vi "AI@SegmentEditor__Parameter.vi"(1 "ParamterIn":string) -> (0 "ParamterOut":string)   [LabVIEW 2020]
uses:
  MainFrame/Global.vi
  <vilib>/vision/NI_Vision_Development_Module.lvlib
panel:
  out "Image":T1(plugin-control)
  in  "Preview":bool
  in  "SubDir":string(combo)
  in  "Capture":string(combo)
  in  "Confirm":bool
  # "AI@SegmentEditor $Capture(\\$Directory)"
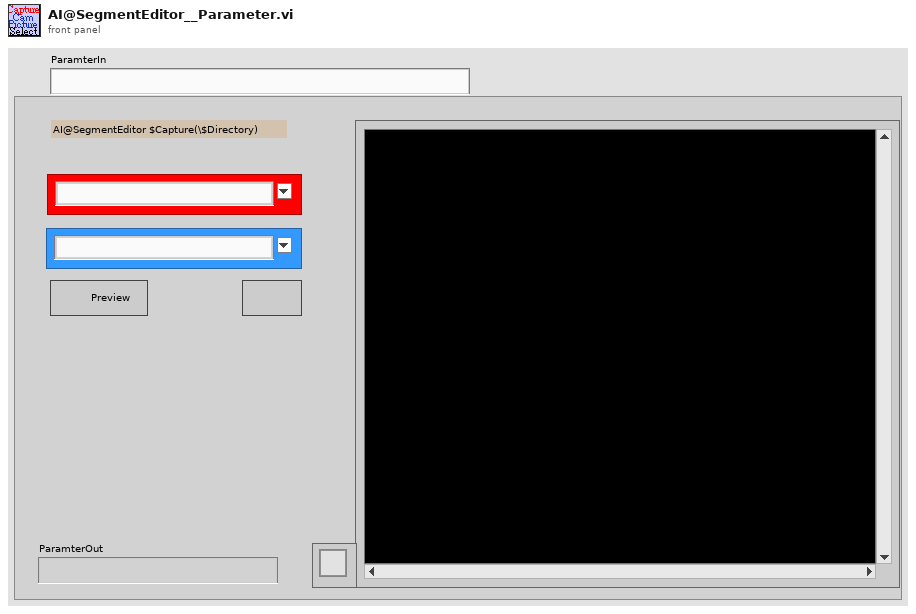
[diagram p1: front panel]
types:
  T1 = typedef "IMAQ Image.ctl" = refnum<image>
  T2 = cluster{"Browser Size":cluster{"X":i32, "Y":i32}, "Images per Line":i32, "Background Color":u32, "Frame Size":i32, "Frame Style":u16}
  T3 = typedef "Image Type" = u32
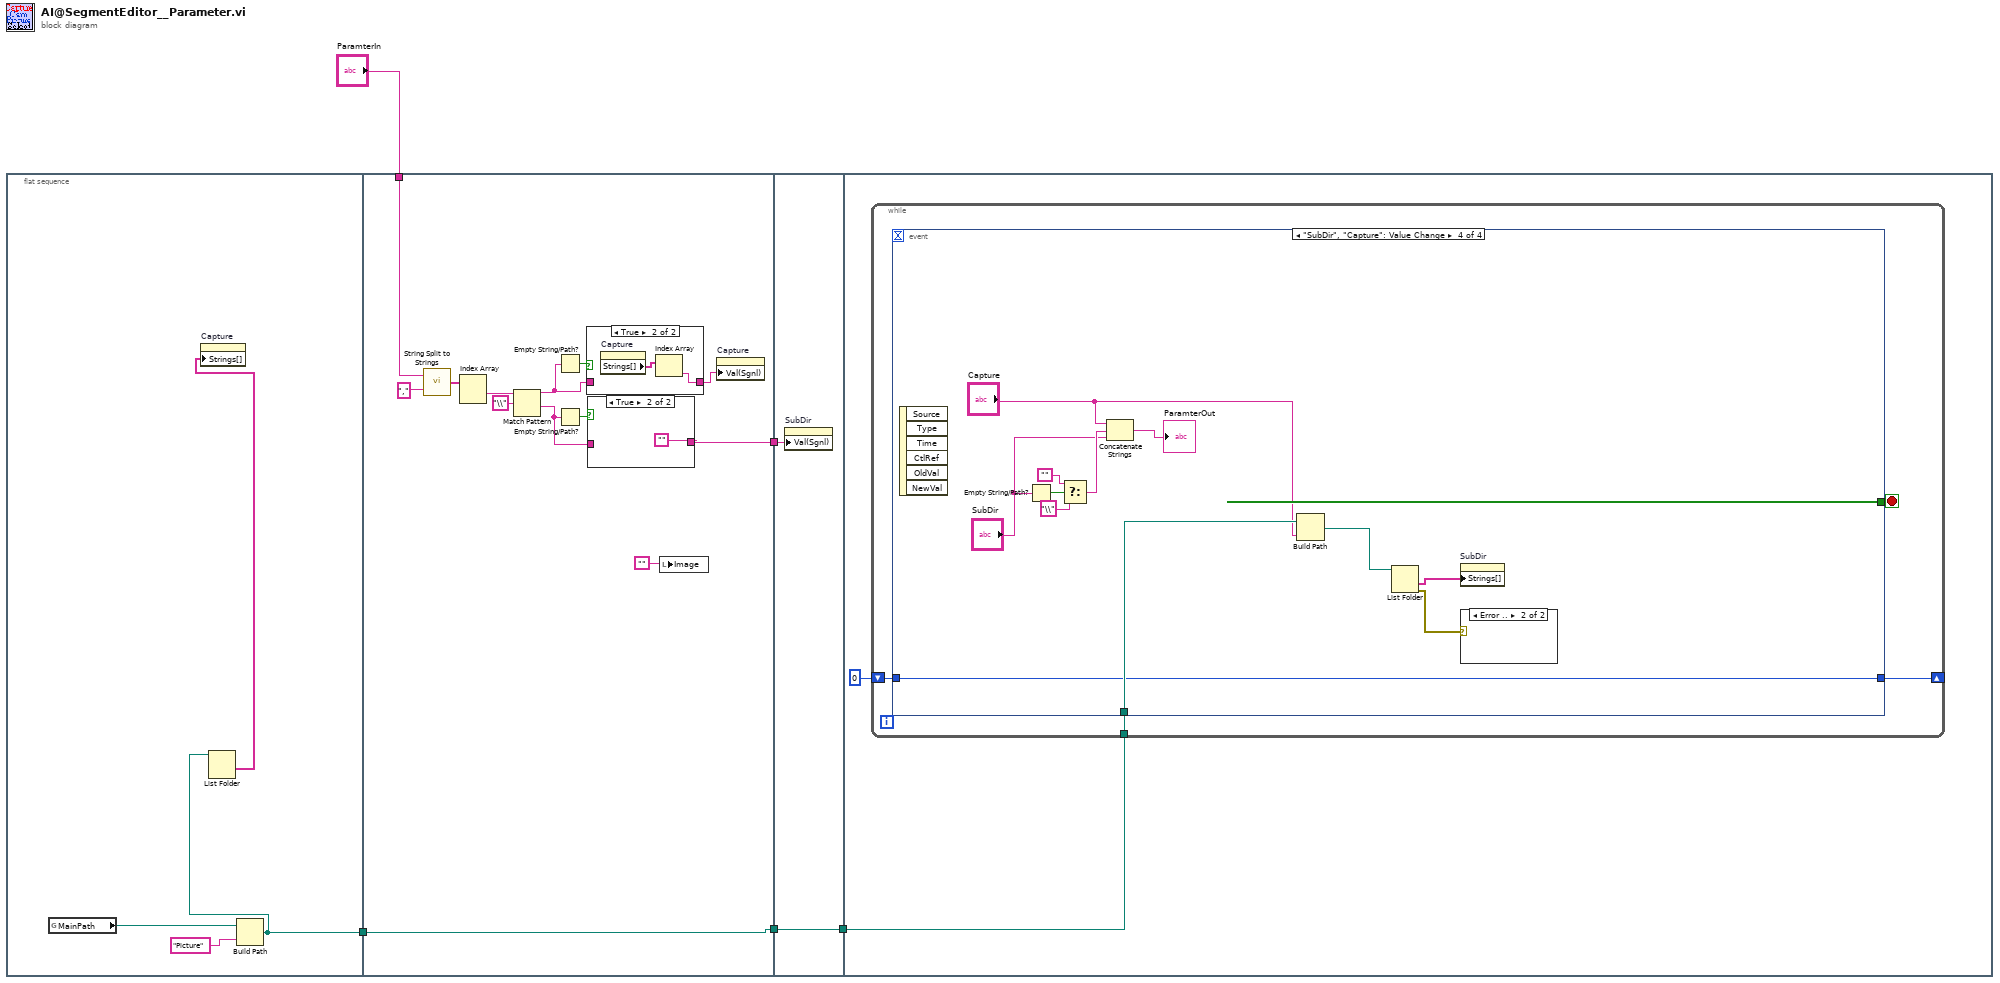
[diagram p0: block diagram]
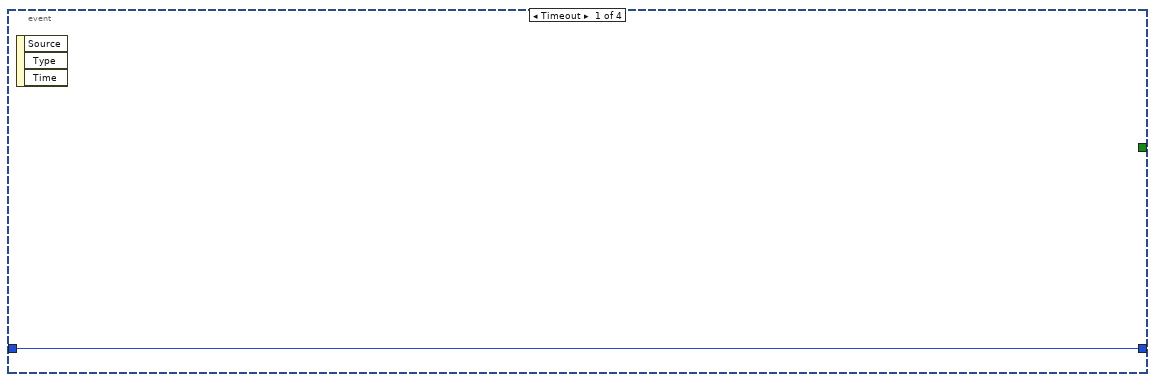
[diagram p4: hidden frame]
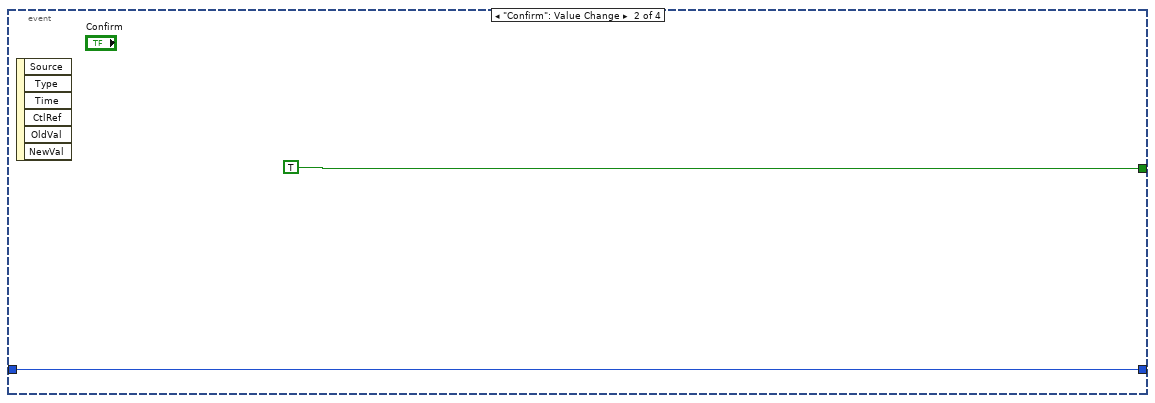
[diagram p5: hidden frame]
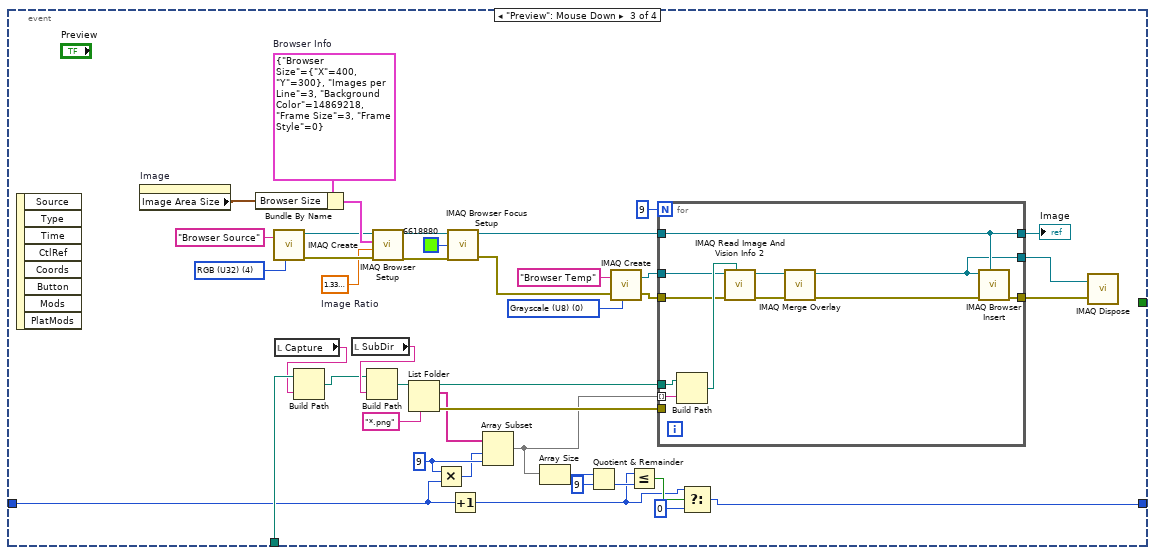
[diagram p6: hidden frame]
diagram:
  n1 = flat-sequence {
    tunnel: [w7] -> w2
    tunnel: "ParamterIn" -> [w20]
    tunnel: [w18] -> w3
    tunnel: w2 -> [w18]
    tunnel: [w17] -> w1
    tunnel: [w29] -> w4
    tunnel: w3 -> [w29]
    tunnel: w1 -> [w28]
    tunnel: w4 -> [w31]
    frame #0 {
      n2 = global read "Global.vi" "MainPath"() -> (w8:path)
      n3 = Build Path(base path=w8, name or relative path="Picture") -> (appended path=w7:path)
      n4 = List Folder(path=w7) -> (folder names=w6:string[])  [unwired: 3 in, 3 out]
      n5 = property on="Capture" class="CmbBox"("Strings[]"=w6) -> ()  [unwired: 2 in, 2 out]
    }
    frame #1 {
      n6 = call "String Split to Strings.vi"("search string/char (-)"=",", "String"=w20) -> ("Array"=w22:string[])
      n7 = Index Array(array=w22) -> (element #1=w14:string)  [unwired: 2 in, 1 out]
      n8 = Match Pattern(string=w14, regular expression="\\") -> (before substring=w12:string, after substring=w11:string)  [unwired: 1 in, 2 out]
      n9 = Empty String/Path?(string/path=w12) -> (empty?=w19:bool)
      n10 = Empty String/Path?(string/path=w11) -> (empty?=w15:bool)
      n11 = case shown="True" w19 {
        tunnel: w12 -> [w25 _]
        tunnel: [w25 w26] -> w16
        frame False {
        }
        frame True {
          n12 = property on="Capture" class="CmbBox"() -> ("Strings[]"=w27:string[])  [unwired: 2 in, 2 out]
          n13 = Index Array(array=w27) -> (element=w26:string)  [unwired: 1 in]
        }
      }
      n14 = case shown="True" w15 {
        tunnel: [w23 ""] -> w17
        tunnel: w11 -> [w23 _]
        frame False {
        }
        frame True {
        }
      }
      n15 = local write "Image"("") -> ()
      n16 = property on="Capture" class="CmbBox"("Val(Sgnl)"=w16) -> ()  [unwired: 2 in, 2 out]
    }
    frame #2 {
      n17 = property on="SubDir" class="CmbBox"("Val(Sgnl)"=w28) -> ()  [unwired: 2 in, 2 out]
    }
    frame #3 {
      n18 = while {
        tunnel: w31 -> [w34]
        shift-right: [w32] -> _
        shift-left: 0 -> [w33]
        stop <- w35 stop-if-true
        n19 = event shown="[3] \"SubDir\", \"Capture\": Value Change" {
          selector: _ -> [_ _ _ _]
          dyn-events: _ -> [_ _ _ _]
          timeout: _ -> [_ _ _ _]
          tunnel: [_ TRUE _ _] -> w35
          tunnel: w34 -> [_ _ w54 w100]
          tunnel: w33 -> [w36 w37 w48 w91]
          tunnel: [w36 w37 w40 w91] -> w32
          event Timeout {
            n20 = event-data() -> ()  [unwired: 1 in, 3 out]
          }
          event "Confirm": Value Change {
            n21 = event-data() -> ()  [unwired: 1 in, 6 out]
          }
          event "Preview": Mouse Down {
            w50 = 9 ("length")
            w58 = sgl 1.33  # Image Ratio
            w75 = T2 {"Browser Size"={"X"=400, "Y"=300}, "Images per Line"=3, "Background Color"=14869218, "Frame Size"=3, "Frame Style"=0}  # Browser Info
            w66 = T3 0 items=["Grayscale (U8)", "Grayscale (I16)", "Grayscale (SGL)", "Complex (CSG)", "RGB (U32)", "HSL (U32)", "RGB (U64)", "Grayscale (U16)"] ("Image Type")
            w64 = T3 4 items=["Grayscale (U8)", "Grayscale (I16)", "Grayscale (SGL)", "Complex (CSG)", "RGB (U32)", "HSL (U32)", "RGB (U64)", "Grayscale (U16)"] ("Image Type")
            n22 = event-data() -> ()  [unwired: 1 in, 8 out]
            n23 = property on="Image" class="ImageControl"() -> ("Image Area Size"=w76:cluster{"Width":u32, "Height":u32})  [unwired: 2 in, 2 out]
            n24 = Bundle By Name(cluster=w75, "Browser Size"=w76) -> (w77:T2)
            n25 = call "IMAQ Create"("Image Name"="Browser Source", "Image Type"=w64) -> ("New Image"=w62:T1, "error out"=w63:errorcluster)  [unwired: 3 in]
            n26 = local read "Capture"() -> (w53:string)
            n27 = Build Path(base path=w54, name or relative path=w53) -> (appended path=w52:path)
            n28 = local read "SubDir"() -> (w57:string)
            n29 = Build Path(base path=w52, name or relative path=w57) -> (appended path=w56:path)
            n30 = call "IMAQ Browser Setup"("error in (no error)"=w63, "Image Ratio"=w58, "Browser Info"=w77, "Image In"=w62) -> ("error out"=w71:errorcluster, "Image Browser Out"=w70:T1)  [unwired: 2 out]
            n31 = List Folder(path=w56, pattern="*.png") -> (path out=w61:path, filenames=w39:string[], error out=w78:errorcluster)  [unwired: 2 in, 1 out]
            n32 = Multiply(x=w50, y=w48) -> (x*y=w49:i32)
            n33 = call "IMAQ Browser Focus Setup"("error in (no error)"=w71, "Focus Color"=u32 6618880, "Image Browser In"=w70) -> ("error out"=w73:errorcluster, "Image Browser Out"=w72:T1)  [unwired: 1 in]
            n34 = Increment(x=w48) -> (x+1=w42:i32)
            n35 = Array Subset(array=w39, index=w49, length=w50) -> (w47:string[])
            n36 = Array Size(array=w47) -> (size(s)=w46:i32)
            n37 = Quotient & Remainder(x=w46, y=9) -> (floor(x/y)=w44:i32)  [unwired: 1 out]
            n38 = call "IMAQ Create"("Image Name"="Browser Temp", "Image Type"=w66, "error in (no error)"=w73) -> ("New Image"=w68:T1, "error out"=w59:errorcluster)  [unwired: 2 in]
            n39 = Less Or Equal?(x=w42, y=w44) -> (x <= y?=w43:bool)
            n40 = for {
              N: 9 -> [_]
              tunnel: w72 -> [w85]
              tunnel: w61 -> [w90]
              tunnel: w59 -> [w88]
              tunnel: [w87] -> w60
              tunnel: [w85] -> w79
              tunnel: w68 -> [w86]
              tunnel: [w82] -> w69
              tunnel: w78 -> [_]
              tunnel: w47 -> [w80] mode=indexing
              n41 = Build Path(base path=w90, name or relative path=w80) -> (appended path=w89:path)
              n42 = call "IMAQ Read Image And Vision Info 2"("File Path"=w89, "error in (no error)"=w88, "Image"=w86) -> ("error out"=w84:errorcluster, "Image Out"=w83:T1)  [unwired: 6 in, 1 out]
              n43 = call "IMAQ Merge Overlay"("error in (no error)"=w84, "Image Src"=w83) -> ("error out"=w81:errorcluster, "Image Dst Out"=w82:T1)  [unwired: 8 in]
              n44 = call "IMAQ Browser Insert"("Image Browser In"=w85, "error in (no error)"=w81, "Image to Add"=w82) -> ("error out"=w87:errorcluster)  [unwired: 4 in, 4 out]
            }
            "Image" <- w79
            n45 = Select(t=w42, s=w43, f=0) -> (s? t:f=w40:i32)
            n46 = call "IMAQ Dispose"("Image"=w69, "error in (no error)"=w60) -> ()  [unwired: 4 in, 1 out]
          }
          event "SubDir", "Capture": Value Change {
            n47 = event-data() -> ()  [unwired: 1 in, 6 out]
            n48 = Empty String/Path?(string/path="SubDir") -> (empty?=w96:bool)
            n49 = Select(t="", s=w96, f="\\" ("string")) -> (s? t:f=w93:string)
            n50 = Concatenate Strings("Capture", w93, "SubDir") -> (→"ParamterOut":string)
            n51 = Build Path(base path=w100, name or relative path="Capture") -> (appended path=w99:path)
            n52 = List Folder(path=w99) -> (folder names=w98:string[], error out=w101:errorcluster)  [unwired: 3 in, 2 out]
            n53 = property on="SubDir" class="CmbBox"("Strings[]"=w98) -> ()  [unwired: 2 in, 2 out]
            n54 = case shown="Error .." w101 {
              frame No Error {
              }
              frame Error {
              }
            }
          }
        }
      }
    }
  }
